vi "WakerControl.vi"(6 "Button 4":bool, 7 "Button 2":bool, 8 "Button 3":bool, 9 "Button 1":bool) -> (2 "Speed Out":dbl)   [LabVIEW 2012]
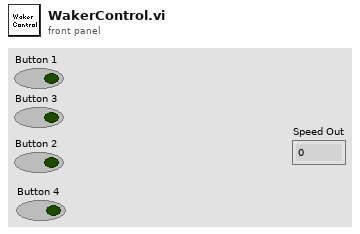
[diagram p1: front panel]
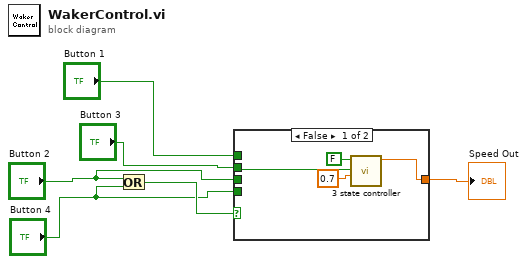
[diagram p0: block diagram]
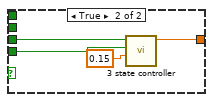
[diagram p2: hidden frame]
diagram:
  n1 = Or(x="Button 2", y="Button 4") -> (x .or. y?=w6:bool)
  n2 = case shown="False" w6 {
    tunnel: "Button 2" -> [_ w14]
    tunnel: "Button 4" -> [_ w13]
    tunnel: [w9 w11] -> w5
    tunnel: "Button 3" -> [w7 _]
    tunnel: "Button 1" -> [_ _]
    frame False {
      n3 = call "3 state controller.vi"("Power"=0.7, "Backward"=w7, "Forward"=FALSE) -> ("Numeric"=w9:dbl)  [unwired: 8 in]
    }
    frame True {
      n4 = call "3 state controller.vi"("Power"=0.15, "Backward"=w13, "Forward"=w14) -> ("Numeric"=w11:dbl)  [unwired: 8 in]
    }
  }
  "Speed Out" <- w5
